vi "main.vi"() -> ()   [LabVIEW 2025]
panel:
  out "element":dbl
  out "Running?":i32
  in  "stop":bool
  # "This main VI is just running an empty, timed while loop.\nKeep this exe running to execute VIs in it's context."
  # "Additionally there is queue of type double that waits\nfor a value to be sent. If received, it will be displayed below\nwith a timestamp.\nUse the Send-To-Queue.py (calls sendqueue.vi) to send\na random number to that queue."
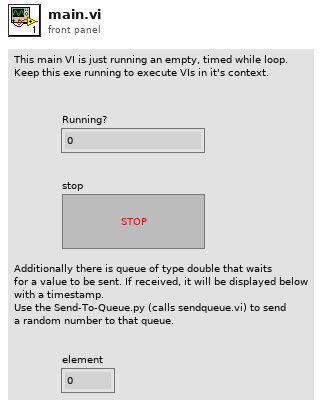
[diagram p1: front panel]
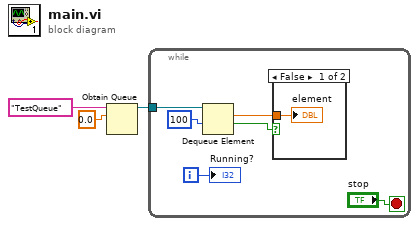
[diagram p0: block diagram]
diagram:
  n1 = Obtain Queue(name (unnamed)="TestQueue", element data type=0.0) -> (queue out=w1:refnum<queue>)  [unwired: 3 in, 2 out]
  n2 = while {
    tunnel: w1 -> [w6]
    i -> [w8]
    stop <- "stop" stop-if-true
    n3 = Dequeue Element(queue=w6, timeout in ms (-1)=100) -> (element=w7:dbl, timed out?=w4:bool)  [unwired: 1 in, 2 out]
    n4 = case shown="False" w4 {
      tunnel: w7 -> [w10 _]
      frame False {
        "element" <- w10
      }
      frame True {
      }
    }
    "Running?" <- w8
  }
